vi "dfd_Direct_IIR_I_C.vi"() -> ()   [LabVIEW 2017, in "NI_DigFilterTemp.lvlib"]
uses:
  <vilib>/addons/Digital Filter Design/NI_DigFilterTemp.lvlib
panel:
  in  "String":string="\n\n/* ---- Constants ----*/\n#define %CapName%_N_XSTATES %kXStatesAmt%\n#define %CapName%_N_YSTATES %kYStatesAmt%\n#define %CapName%_N_STATES (%CapName%_N_XSTATES + %CapName%_N_YSTATES)\n#define %CapName%_N_COEFA %CapName%_N_YSTATES\n#define %CapName%_N_COEFB %CapName%_N_XSTATES\n\n/* ---- Global Variables Declaration ----*/\nstatic %CoefAType% %FilterBlkName%_CoefA[%CapName%_N_COEFA];\nstatic %CoefBType% %FilterBlkName%_CoefB[%CapName%_N_COEFB];\n%InternalFunctionsDeclaration%\n\n%ShiftDefine%\n\n%AssistantFunctions%\n\n/* ---- Implement the Fixed-Point Filter ---- */\n%OutType% %FilterBlkName%_Filtering (%InType% sampleIn, %FilterBlkName%_State state)\n{\n\tI32 accA;\n\t%FilterBlkName%_State xstate = state;\n\t%FilterBlkName%_State ystate = state + %CapName%_N_XSTATES;\n\tint i;\n\n\t/* Update the internal states */\n\txstate[0] = sampleIn;\n\n\t/* Filtering */\n\taccA = 0;\n\tfor (i = (%CapName%_N_COEFB-1); i >= 0; i--)\n\t{\n\t\taccA += (%FilterBlkName%_%MultB%((%InType%)xstate[i], %FilterBlkName%_CoefB[i]) << PROD2SUM);\n\t\txstate[i] = (i==0) ? 0 : xstate[i-1];\n\t}\n\n\tfor (i = (%CapName%_N_COEFA-1); i >= 0; i--)\n\t{\n\t\taccA -= (%FilterBlkName%_%MultA%(%PreMultCast%(ystate[i] << DELAY2MULT), %FilterBlkName%_CoefA[i]) << PROD2SUM);\n\t\tystate[i] = (i==0) ? 0 : ystate[i-1];\n\t}\n\n\t/* Update the internal states */\n\tystate[0] = (accA << SUM2DELAY);\n\n\t%ApplyGainAccA%\n\n\treturn (%OutType%)accA;\n}\n\n/* ---- Internal Functions ---- */\n%InternalFunctions%\n\n/* ---- Filter Coefficients ---- */\nstatic %CoefAType% %FilterBlkName%_CoefA [] = {\n%CoefficientsA%\n};\nstatic %CoefBType% %FilterBlkName%_CoefB [] = {\n%CoefficientsB%\n};\n"
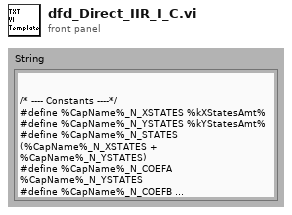
[diagram p1: front panel]
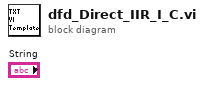
[diagram p0: block diagram]
diagram:
